vi "loop.vi"() -> ()   [LabVIEW 2010]
panel:
  out "current value":string
  in  "Wait/s":dbl format="%.2f"
  in  "Step":dbl format="%.2f"
  out "error out":errorcluster
  in  "error in (no error)":errorcluster
  in  "Stop":dbl format="%.2f"
  in  "Start":dbl format="%.2f"
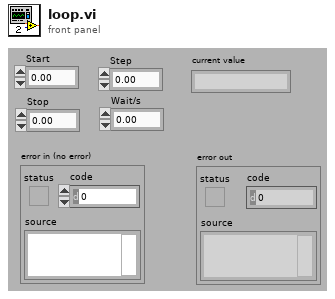
[diagram p1: front panel]
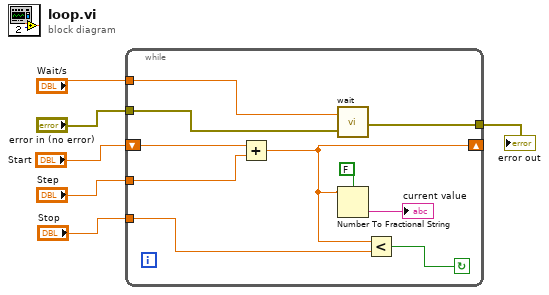
[diagram p0: block diagram]
diagram:
  n1 = while {
    tunnel: "error in (no error)" -> [w8]
    tunnel: [w12] -> w6
    shift-right: [w7] -> _
    shift-left: "Start" -> [w14]
    tunnel: "Step" -> [w16]
    tunnel: "Stop" -> [w15]
    tunnel: "Wait/s" -> [w11]
    stop <- w13 continue-if-true
    n2 = Add(x=w14, y=w16) -> (x+y=w7:dbl)
    n3 = call "wait.vi"("error in"=w8, "Wartezeit in Sek"=w11) -> ("error out"=w12:errorcluster)  [unwired: 1 in]
    n4 = Number To Fractional String(use system decimal point (T)=FALSE, number=w7) -> (F-format string=→"current value":string)  [unwired: 2 in]
    n5 = Less?(x=w7, y=w15) -> (x < y?=w13:bool)
  }
  "error out" <- w6
